vi "LWXPS_PositionerBacklashGet.vi"(8 "LabVIEW error IN":errorcluster, 10 "Positioner Name":string, 11 "XPS Reference IN":refnum<k24>) -> (0 "XPS Error String":string, 1 "Backlask Status":string, 2 "Backlash Value":dbl, 3 "Returned error code":i32, 4 "LabVIEW error OUT":errorcluster, 5 "XPS Reference OUT":refnum<k24>)   [LabVIEW 2014]
uses:
  D:/XPSQ8_LabView_Library/Development/Source/Dll/Newport.XPS.CommandInterface.dll
  Dll/Newport.XPS.CommandInterface.dll
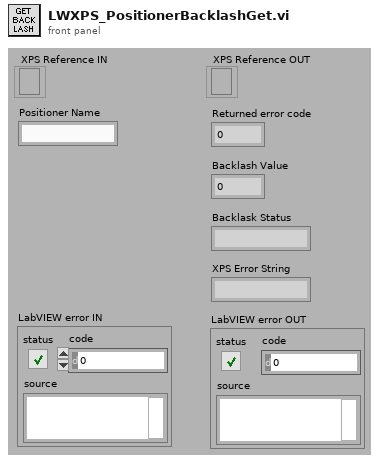
[diagram p1: front panel]
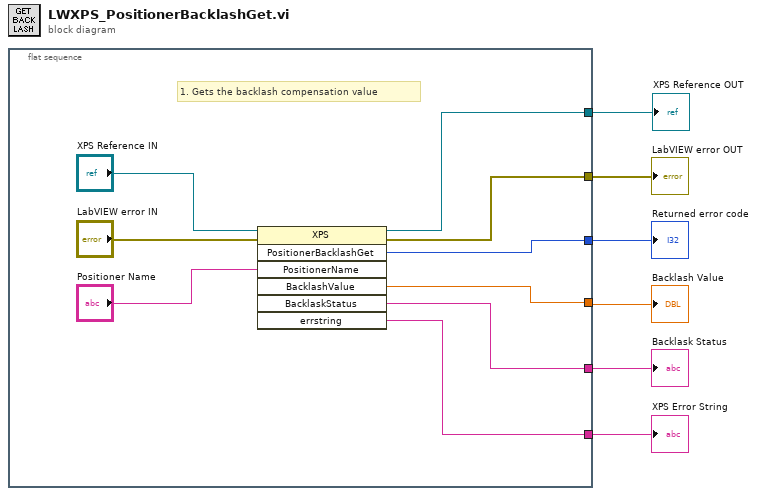
[diagram p0: block diagram]
diagram:
  n1 = flat-sequence {
    tunnel: [w11] -> w6
    tunnel: [w14] -> w5
    tunnel: [w10] -> w4
    tunnel: [w7] -> w3
    tunnel: [w9] -> w2
    tunnel: [w8] -> w1
    frame #0 {
      # "1. Gets the backlash compensation value"
      n2 = invoke class="XPS" method="PositionerBacklashGet"(reference="XPS Reference IN", error in="LabVIEW error IN", "PositionerName"="Positioner Name") -> (reference out=w11:refnum<k24>, error out=w14:errorcluster, "PositionerBacklashGet"=w10:i32, "BacklashValue"=w9:dbl, "BacklaskStatus"=w8:string, "errstring"=w7:string)  [unwired: 4 in, 1 out]
    }
  }
  "XPS Error String" <- w3
  "XPS Reference OUT" <- w6
  "LabVIEW error OUT" <- w5
  "Returned error code" <- w4
  "Backlash Value" <- w2
  "Backlask Status" <- w1
